vi "Result to Trace.vi"(8 "error in (no error)":errorcluster, 10 "Result":string[][](array[string]), 11 "Data.PGQL in":refnum<class "LV-Data.PGSQL.lvclass">) -> (0 "error out":errorcluster, 2 "Cluster":cluster{timestamp[], dbl[]}, 3 "Data.PGSQL out":refnum<class "LV-Data.PGSQL.lvclass">)   [LabVIEW 2019, in "LV-Data.PGSQL.lvclass"]
uses:
  LV-Data.PGSQL.lvclass
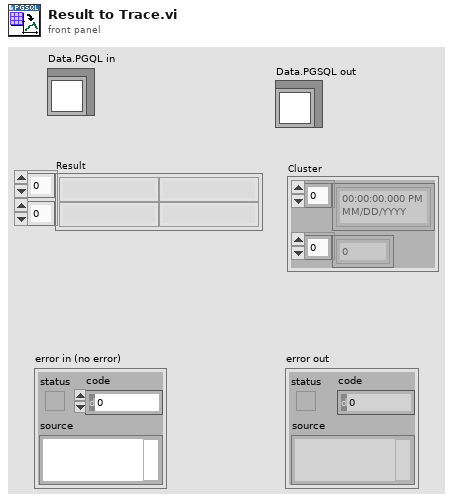
[diagram p1: front panel]
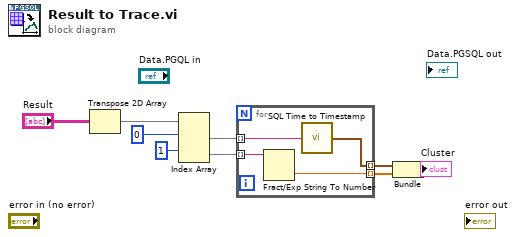
[diagram p0: block diagram]
diagram:
  n1 = Transpose 2D Array(2D array="Result") -> (transposed array=w7:string[][])
  n2 = Index Array(array=w7, index (row) #1=0 ("index (row)"), index (row) #2=1 ("index (row)")) -> (element #1=w4:string[], element #2=w3:string[])  [unwired: 2 in]
  n3 = for {
    tunnel: w4 -> [w13] mode=indexing
    tunnel: w3 -> [w12] mode=indexing
    tunnel: [w11] -> w1 mode=indexing
    tunnel: [w10] -> w2 mode=indexing
    n4 = Fract/Exp String To Number(string=w12) -> (number=w11:dbl)  [unwired: 3 in, 1 out]
    n5 = call "SQL Time to Timestamp.vi"("date/time string"=w13) -> ("Time Stamp"=w10:timestamp)
  }
  n6 = Bundle(w2, w1) -> (→"Cluster":cluster{timestamp[], dbl[]})  [unwired: 1 in]
